vi "2_AdvancedDemo_TH260Histo.vi"() -> ()   [LabVIEW 2010]
uses:
  Types/TH260_UIThread_Cmds.ctl
  Types/TH260_UIThread_Data.ctl
  Types/TH260_InputChannel.ctl
  <vilib>/Utility/error.llb/DialogType.ctl
  _lib/PQ/TimeHarp260/th260lib_x86_x64_UIThread.llb/TH260_DllPath_global.vi
  _lib/PQ/TimeHarp260/TH260_LibVersion_global.vi
  _lib/PQ/TimeHarp260/TH260_InitInfo.ctl
  _lib/PQ/TimeHarp260/TH260_MeasMode.ctl
  _lib/PQ/TimeHarp260/TH260_TimingMode.ctl
panel:
  in  "Settings":bool=TRUE
  in  "Run continuously":bool=TRUE caption="Conti."
  in  "Start":bool
  in  "Scale":bool
  out "CountRates":i32[](graph)
  in  "HistoLength":i32(ring)=6 caption="Num Bins" items=["1024", "2048", "4096", "8192", "16384", "32768"]
  in  "OvlLevel":u32=100000 caption="Ovl.Level" min=1 step=1
  in  "StopOvl.":bool=TRUE
  in  "AcqTime":i32=1000 caption="Acqu.     ms" min=1 max=360000000 step=1
  in  "Binning":i32(ring) caption="Resol.      ps" items=["25", "50", "100", "200", "400", "800", "1600", "3200", "6400", "12800", "25600", "51200", "102400", "204800", "409600", "819200", "1638400", "3276800", "6553600", "13107200", "26214400", "52428800"]
  in  "HistoOffset":i32 caption="Offset      ns" min=0 max=100000000 step=1
  out "HistoGraph":T1(graph)={0.0, "Resolution"=0.001, "Histogram"=array8x1024[8192 elements]}
  in  "SyncTrgEdge":i32(ring) caption="Edge" items=["falling", "rising"]
  in  "SyncTrgLevel":i32=-100 caption="Level        mV" min=-1200 max=1200 step=1
  in  "SyncCFDLevel":i32=-100 caption="Level        mV" min=-1200 max=0 step=1
  in  "SyncZeroX":i32=-10 caption="ZeroCr.    mV" min=-40 max=0 step=1
  in  "SyncDivider":i32(ring)=3 caption="Divider" items=["1", "2", "4", "8"]
  in  "SyncOffset":i32 caption="Offset        ps" min=-99999 max=99999 step=1
  in  "Channels":T2[](array[typedef])=[{"Name"="Inp.Chan 1", "Enable"=TRUE, "Offset"=0, "CFDLevel"=50, "ZeroX"=10, "dtcode"=0, "TrgLevel"=-100, "TrgEdge"=0}, {"Name"="Inp.Chan 2", "Enable"=TRUE, "Offset"=0, "CFDLevel"=50, "ZeroX"=10, "dtcode"=0, "TrgLevel"=-100, "TrgEdge"=0}, {"Name"="Inp.Chan 3", "Enable"=TRUE, "Offset"=0, "CFDLevel"=50, "ZeroX"=10, "dtcode"=0, "TrgLevel"=-100, "TrgEdge"=0}, {"Name"="Inp.Chan 4", "Enable"=TRUE, "Offset"=0, "CFDLevel"=50, "ZeroX"=10, "dtcode"=0, "TrgLevel"=-100, "TrgEdge"=0}, {"Name"="Inp.Chan 5", "Enable"=TRUE, "Offset"=0, "CFDLevel"=50, "ZeroX"=10, "dtcode"=0, "TrgLevel"=-100, "TrgEdge"=0}, {"Name"="Inp.Chan 6", "Enable"=TRUE, "Offset"=0, "CFDLevel"=50, "ZeroX"=10, "dtcode"=0, "TrgLevel"=-100, "TrgEdge"=0}, {"Name"="Inp.Chan 7", "Enable"=TRUE, "Offset"=0, "CFDLevel"=50, "ZeroX"=10, "dtcode"=0, "TrgLevel"=-100, "TrgEdge"=0}, {"Name"="Inp.Chan 8", "Enable"=TRUE, "Offset"=0, "CFDLevel"=50, "ZeroX"=10, "dtcode"=0, "TrgLevel"=-100, "TrgEdge"=0}] {"TrgEdge" items=["falling", "rising"]; "TrgLevel" min=-1200 max=1200 step=1; "dtcode" items=["24", "44", "66", "88", "112", "135", "160", "180"]; "ZeroX" min=-40 max=0 step=1; "Offset" min=-99999 max=99999 step=1; "CFDLevel" min=-1200 max=0 step=1}
  out "SyncRate":string="Sync Rate: 0 cps\n"
  out "OverFlow":bool caption="Overflow:"
  out "Status":string="Initialized!"
  # "Histogram"
  # "Sync"
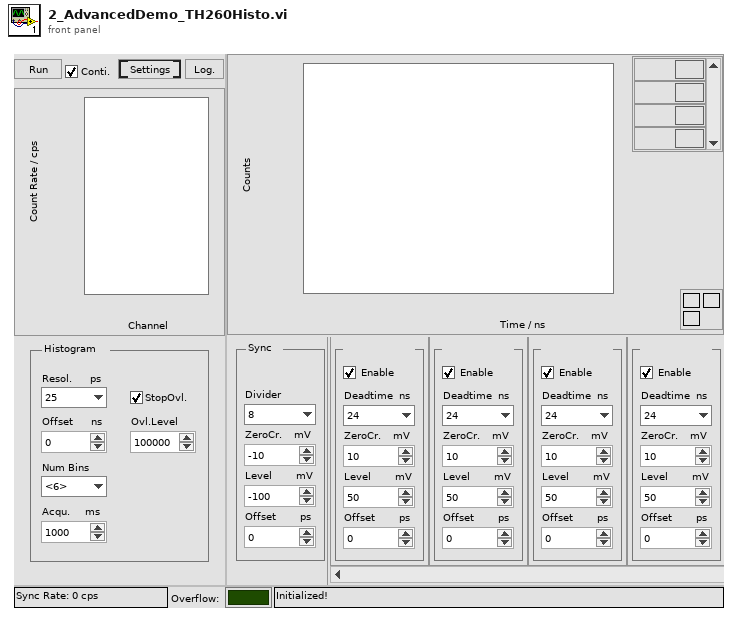
[diagram p1: front panel]
types:
  T1 = cluster{dbl, "Resolution":dbl, "Histogram":u32[][]}
  T2 = typedef "TH260_InputChannel.ctl" = cluster{"Name":string, "Enable":bool, "Offset":i32, "CFDLevel":i32, "ZeroX":i32, "dtcode":i32, "TrgLevel":i32, "TrgEdge":i32}
  T3 = typedef "TH260_UIThread_Data.ctl" = cluster{"Init Info":T4, "DevIdx":i32, "Channels":T2[], "CurrentChannels":i32[], "AcqTime":i32, "Binning":i32, "HistoOffset":i32, "HistoLen":i32, "StopOvl.":bool, "OvlLevel":u32, "StartMeas":bool, "HistoLength":i32, "Resolution":dbl, "Run cont.":bool, "Status":string, "SyncRate":i32, "BitShift":i32, "HistoAcqTime":dbl, "SyncTrgEdge":i32, "SyncTrgLevel":i32, "SyncCFDLevel":i32, "SyncZeroX":i32, "SyncDivider":i32, "SyncOffset":i32}
  T4 = typedef "TH260_InitInfo.ctl" = cluster{"Library Version":string, "Serial No.":string, "Model":string, "Partnum":string, "Version":string, "features":i32, "nchannels":i32, "Base Resolution":dbl, "Bin Steps":i32}
  T5 = typedef "TH260_UIThread_Cmds.ctl" = enum16{"Idle", "Init", "SetInpChanEnable", "SetInpChanOffset", "SetInpChanCFD", "SetInpChanTrg", "SetInpChanDeadtime", "SetSyncDivider", "SetSyncCFD", "SetSyncTrg", "SetSyncOffset", "SetBinning", "SetHistoOffset", "SetHistoLen", "SetStopOvl", "SetBitShift", "SetHistoAcqTime", "GetRates", "StartMeas", "StopMeas", "AbortMeas", "GetResolution", "GetHisto", "ReadFiFo", "WriteStatus", "Resize", "EnableControls", "DisableControls", "Error", "Exit"}
  T6 = enum8{"Enabled", "Disabled", "Disabled and Grayed Out"}
  T7 = typedef "TH260_TimingMode.ctl" = i32
  T8 = typedef "TH260_MeasMode.ctl" = i32
  T9 = typedef "DialogType.ctl" = u16
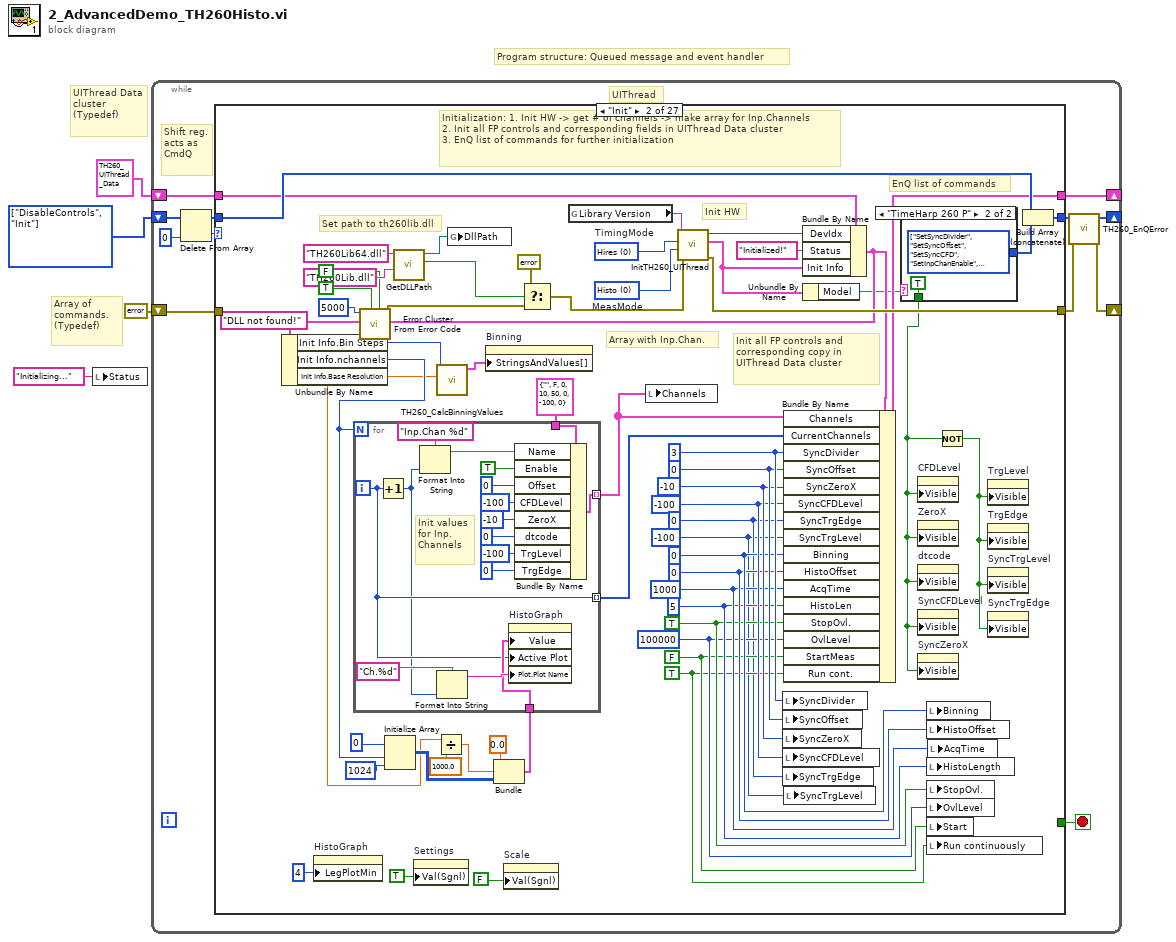
[diagram p0: block diagram]
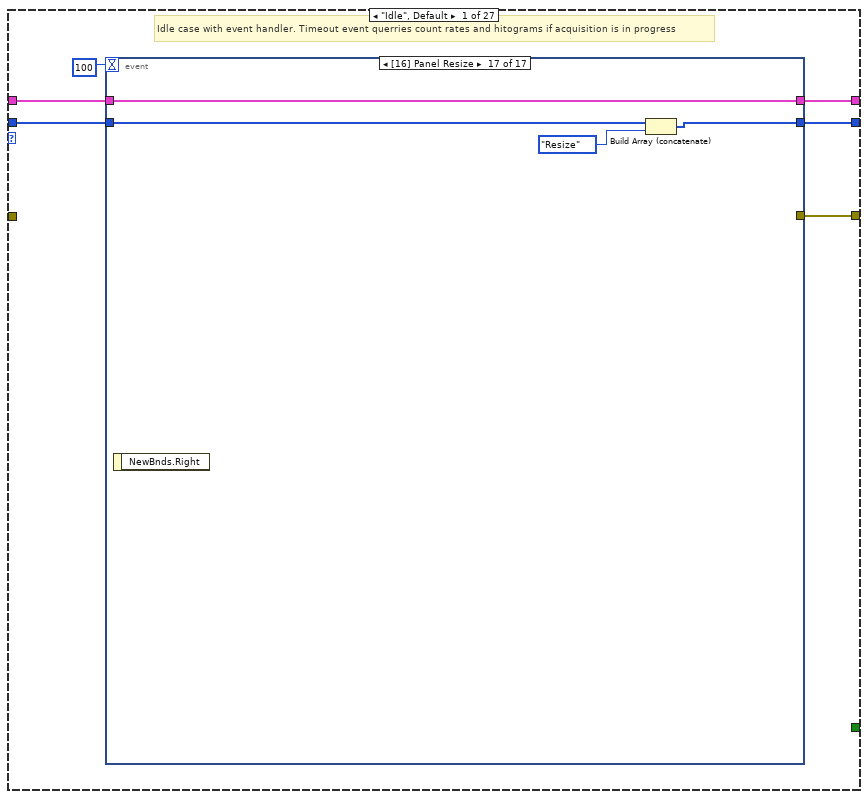
[diagram p2: hidden frame]
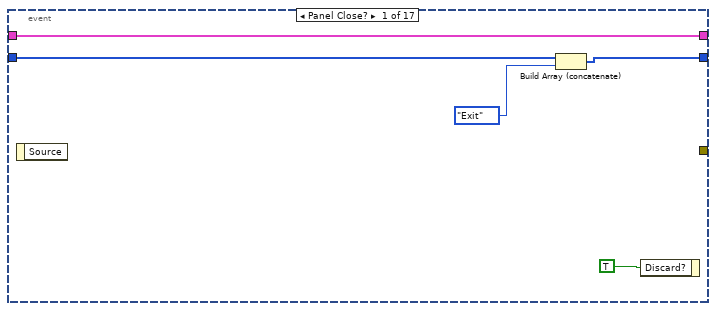
[diagram p3: hidden frame]
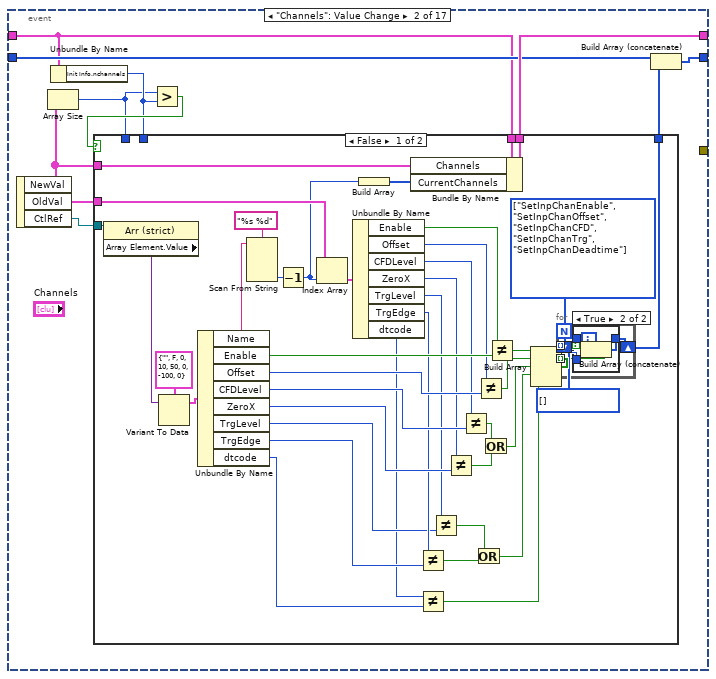
[diagram p4: hidden frame]
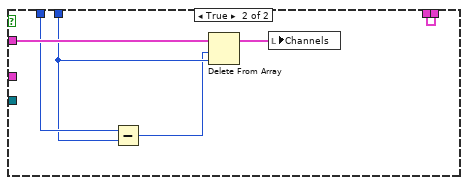
[diagram p6: hidden frame]
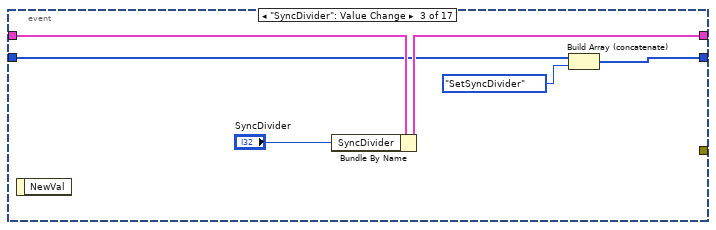
[diagram p7: hidden frame]
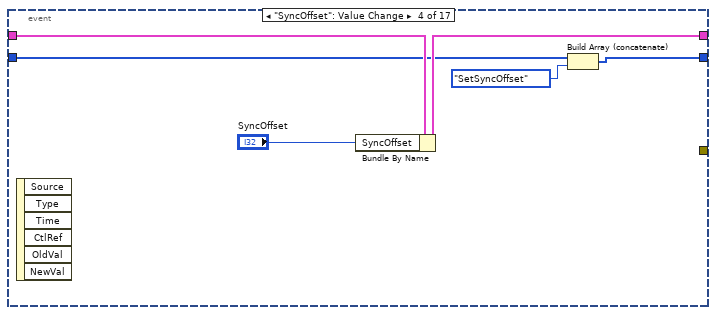
[diagram p8: hidden frame]
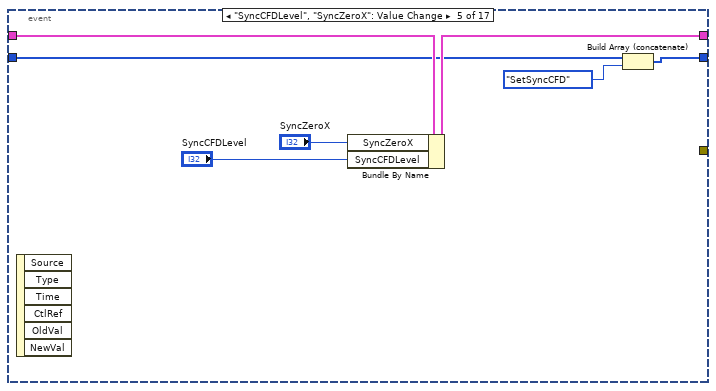
[diagram p9: hidden frame]
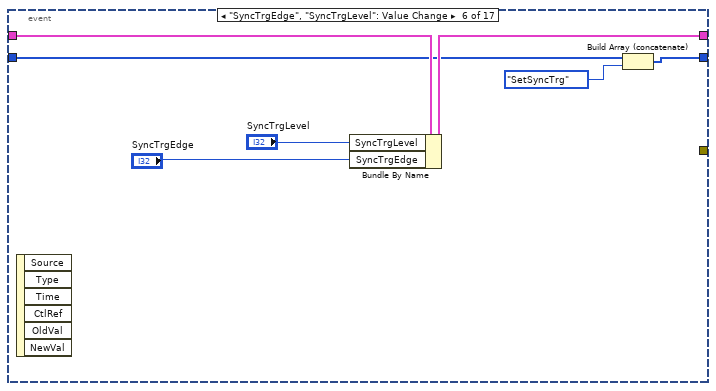
[diagram p10: hidden frame]
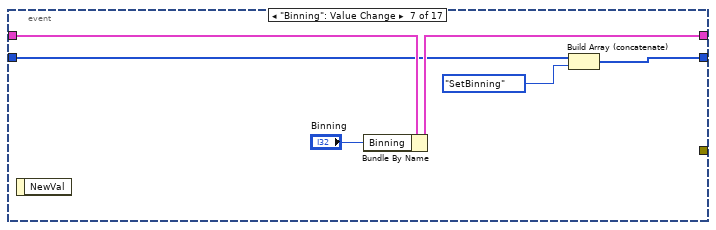
[diagram p11: hidden frame]
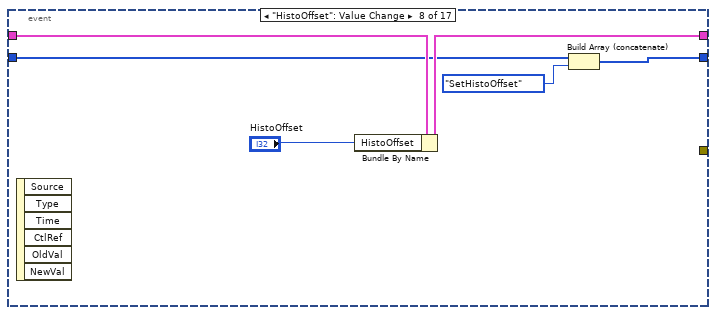
[diagram p12: hidden frame]
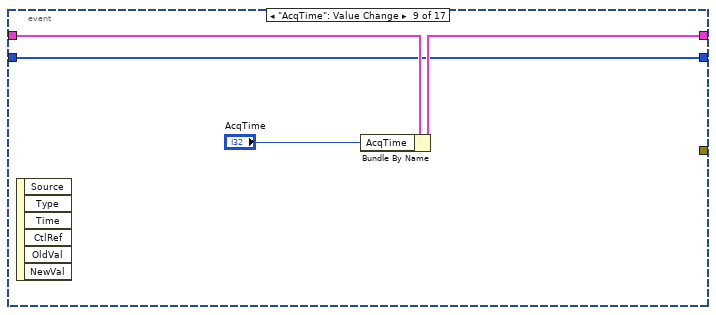
[diagram p13: hidden frame]
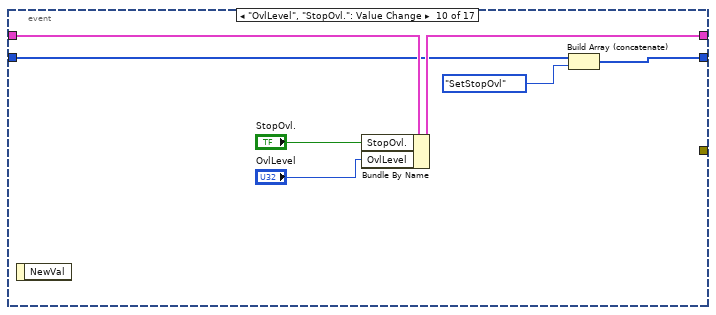
[diagram p14: hidden frame]
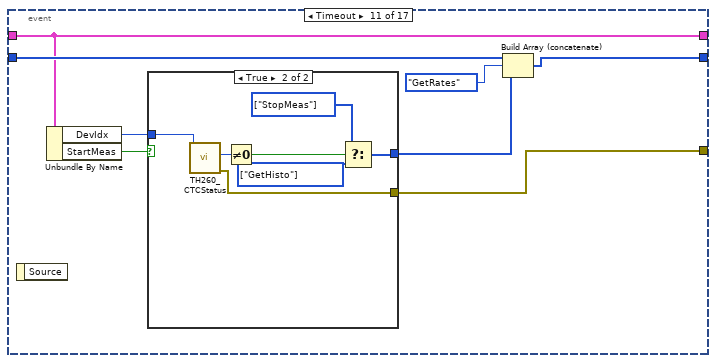
[diagram p15: hidden frame]
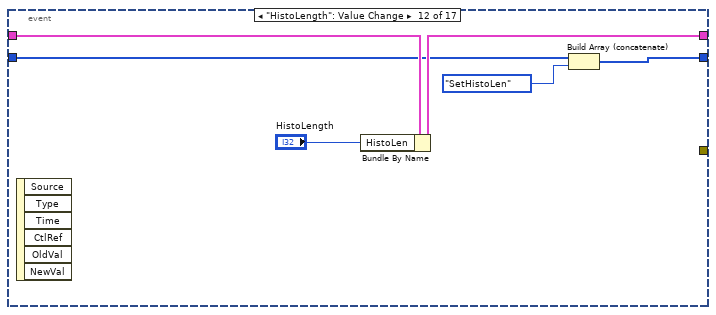
[diagram p17: hidden frame]
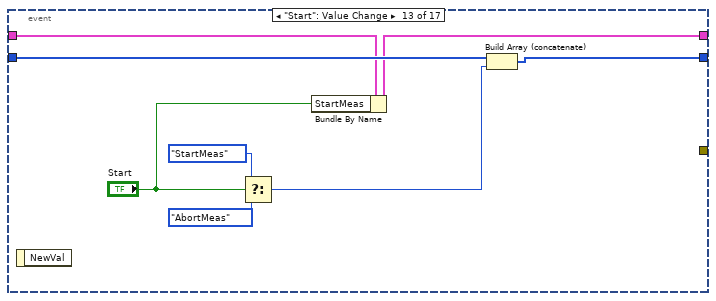
[diagram p18: hidden frame]
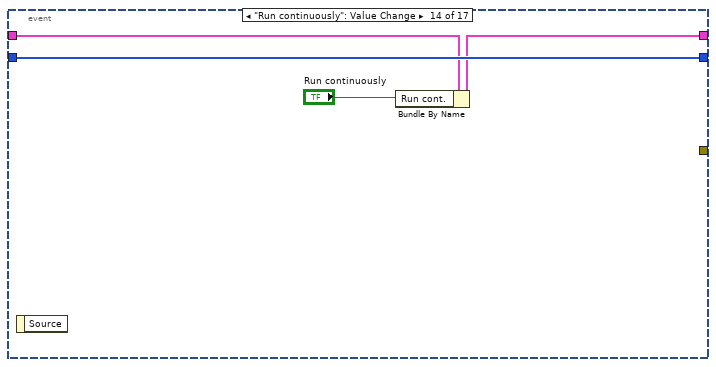
[diagram p19: hidden frame]
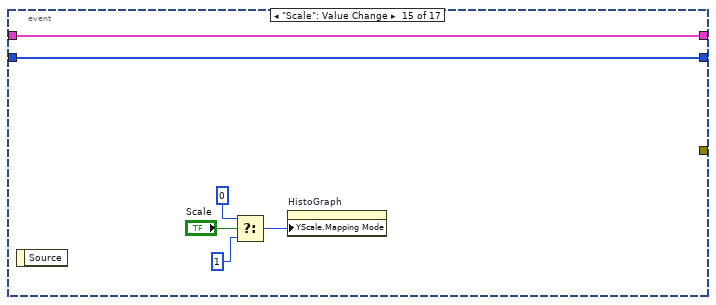
[diagram p20: hidden frame]
diagram:
  w3 = T5[] [enum."DisableControls", enum."Init"] items=["Idle", "Init", "SetInpChanEnable", "SetInpChanOffset", "SetInpChanCFD", "SetInpChanTrg", "SetInpChanDeadtime", "SetSyncDivider", "SetSyncCFD", "SetSyncTrg", "SetSyncOffset", "SetBinning", "SetHistoOffset", "SetHistoLen", "SetStopOvl", "SetBitShift", "SetHistoAcqTime", "GetRates", "StartMeas", "StopMeas", "AbortMeas", "GetResolution", "GetHisto", "ReadFiFo", "WriteStatus", "Resize", "EnableControls", "DisableControls", "Error", "Exit"]
  # "Array of commands.\n(Typedef)"
  # "Program structure: Queued message and event handler"
  # "UIThread Data cluster\n(Typedef)"
  n1 = local write "Status"("Initializing..." ("Status")) -> ()
  n2 = while {
    shift-right: [w5] -> _
    shift-left: w3 -> [w12]
    shift-right: [w15] -> _
    shift-left: T3 {"Init Info"={"Library Version"="", "Serial No."="", "Model"="", "Partnum"="", "Version"="", "features"=0, "nchannels"=0, "Base Resolution"=0.0, "Bin Steps"=0}, "DevIdx"=0, "Channels"=[], "CurrentChannels"=[], "AcqTime"=1, "Binning"=1, "HistoOffset"=1, "HistoLen"=1024, "StopOvl."=FALSE, "OvlLevel"=1024, "StartMeas"=FALSE, "HistoLength"=0, "Resolution"=0.0, "Run cont."=FALSE, "Status"="", "SyncRate"=0, "BitShift"=0, "HistoAcqTime"=0.0, "SyncTrgEdge"=0, "SyncTrgLevel"=-100, "SyncCFDLevel"=10, "SyncZeroX"=3, "SyncDivider"=3, "SyncOffset"=0} -> [w14]
    shift-right: [w7] -> _
    shift-left: errorcluster {"status"=FALSE, "code"=0, "source"=""} ("error IO") -> [w13]
    stop <- w16 stop-if-true
    # "Shift reg.\nacts as\nCmdQ"
    # "UIThread"
    n3 = Delete From Array(array=w12, index=0) -> (deleted portion=w10:T5, array with subset deleted=w9:T5[])  [unwired: 1 in]
    n4 = case shown="\"Init\"" w10 {
      tunnel: [w22 w256 w284 w298 w312 w327 w342 w358 w367 w373 w375 w382 w390 w398 w403 w415 w430 w438 w452 w466 w493 w518 w531 w538 w550 w556 w560] -> w6
      tunnel: [_ _ _ _ _ _ _ _ _ _ _ _ _ _ _ _ _ _ _ _ _ _ _ _ _ _ TRUE] -> w16
      tunnel: [w21 w236 w287 w301 w315 w330 w345 w360 w368 w374 w379 w386 w391 w393 w404 w414 w436 w441 w455 w462 w492 w517 w519 w537 w549 w557 w563] -> w15
      tunnel: w14 -> [w20 w241 w287 w301 w315 w330 w345 w360 w368 w374 w379 w386 w391 w394 w404 w414 w436 w442 w456 w463 w492 w517 w519 w537 w549 w557 w563]
      tunnel: [w17 w258 w285 w299 w313 w328 w343 w356 w366 w372 w378 w385 w389 w397 w402 w413 w435 w444 w458 w464 w488 _ _ _ _ _ w561] -> w8
      tunnel: w13 -> [_ _ _ _ _ _ _ _ _ _ _ _ _ _ _ _ _ _ _ _ _ _ _ _ _ w558 _]
      tunnel: w9 -> [w19 w257 w284 w298 w312 w327 w342 w358 w367 w373 w375 w381 w390 w398 w403 w415 w431 w439 w453 w466 w493 w518 w531 w538 w550 _ w560]
      frame "Idle", Default {
        # "Idle case with event handler. Timeout event querries count rates and hitograms if acquisition is in progress"
        n5 = event shown="[16] Panel Resize" {
          selector: _ -> [_ _ _ _ _ _ _ _ _ _ _ _ _ _ _ _ _]
          dyn-events: _ -> [_ _ _ _ _ _ _ _ _ _ _ _ _ _ _ _ _]
          timeout: 100 -> [_ _ _ _ _ _ _ _ _ _ _ _ _ _ _ _ _]
          tunnel: [w23 w33 w95 w101 w108 w115 w121 w127 w132 w138 w148 w159 w167 w175 w181 w189 w199] -> w22
          tunnel: [w26 w36 w98 w104 w111 w118 w124 w130 w134 w141 w147 w162 w165 w173 w180 w188 w202] -> w21
          tunnel: w20 -> [w26 w32 w99 w105 w112 w119 w125 w131 w135 w142 w147 w163 w166 w174 w180 w188 w202]
          tunnel: w19 -> [w25 w35 w97 w103 w110 w117 w123 w129 w132 w140 w150 w161 w169 w175 w181 w189 w200]
          tunnel: [_ _ _ _ _ _ _ _ _ _ w143 _ _ _ _ _ _] -> w17
          event Panel Close? {
            n6 = event-data() -> ()  [unwired: 1 in, 1 out]
            n7 = Build Array (concatenate)(w25, TH260_UIThread_Cmds."Exit") -> (w23:T5[])
            n8 = event-data("Discard?"=TRUE) -> ()  [unwired: 1 in, 1 out]
          }
          event "Channels": Value Change {
            n9 = event-data() -> ("NewVal"=w31:T2[], "OldVal"=w37:T2[], "CtlRef"=w38:refnum<vi>)  [unwired: 1 in]
            n10 = Array Size(array=w31) -> (size(s)=w28:i32)
            n11 = Unbundle By Name(w32) -> ("Init Info.nchannels"=w29:i32)
            n12 = Greater?(x=w28, y=w29) -> (0:w30:bool)
            n13 = case shown="False" w30 {
              tunnel: w38 -> [w79 _]
              tunnel: w37 -> [w73 _]
              tunnel: [w56 w93] -> w36
              tunnel: [w54 _] -> w34
              tunnel: w32 -> [w51 w93]
              tunnel: w31 -> [w50 w92]
              tunnel: w29 -> [_ w90]
              tunnel: w28 -> [_ w91]
              frame False {
                w39 = T5[] [] items=["Idle", "Init", "SetInpChanEnable", "SetInpChanOffset", "SetInpChanCFD", "SetInpChanTrg", "SetInpChanDeadtime", "SetSyncDivider", "SetSyncCFD", "SetSyncTrg", "SetSyncOffset", "SetBinning", "SetHistoOffset", "SetHistoLen", "SetStopOvl", "SetBitShift", "SetHistoAcqTime", "GetRates", "StartMeas", "StopMeas", "AbortMeas", "GetResolution", "GetHisto", "ReadFiFo", "WriteStatus", "Resize", "EnableControls", "DisableControls", "Error", "Exit"] ("Array")
                w57 = T5[] [enum."SetInpChanEnable", enum."SetInpChanOffset", enum."SetInpChanCFD", enum."SetInpChanTrg", enum."SetInpChanDeadtime"] items=["Idle", "Init", "SetInpChanEnable", "SetInpChanOffset", "SetInpChanCFD", "SetInpChanTrg", "SetInpChanDeadtime", "SetSyncDivider", "SetSyncCFD", "SetSyncTrg", "SetSyncOffset", "SetBinning", "SetHistoOffset", "SetHistoLen", "SetStopOvl", "SetBitShift", "SetHistoAcqTime", "GetRates", "StartMeas", "StopMeas", "AbortMeas", "GetResolution", "GetHisto", "ReadFiFo", "WriteStatus", "Resize", "EnableControls", "DisableControls", "Error", "Exit"]
                n14 = property class="Arr (strict)"(reference=w79) -> ("Array Element.Value"=w78:variant)  [unwired: 1 in, 2 out]
                n15 = Variant To Data(Variant=w78, type=T2 {"Name"="", "Enable"=FALSE, "Offset"=0, "CFDLevel"=10, "ZeroX"=50, "dtcode"=0, "TrgLevel"=-100, "TrgEdge"=0} ("Channel")) -> (data=w55:cluster{})  [unwired: 1 in, 1 out]
                n16 = Unbundle By Name(w55) -> ("Name"=w76:string, "Enable"=w70:bool, "Offset"=w68:i32, "CFDLevel"=w66:i32, "ZeroX"=w64:i32, "TrgLevel"=w47:i32, "TrgEdge"=w46:i32, "dtcode"=w41:i32)
                n17 = Scan From String(format string="%s %d", input string=w76) -> (output 2=w74:i32)  [unwired: 5 in, 3 out]
                n18 = Decrement(x=w74) -> (x-1=w53:i32)
                n19 = Index Array(array=w73, index=w53) -> (element=w72:T2)
                n20 = Unbundle By Name(w72) -> ("Enable"=w71:bool, "Offset"=w69:i32, "CFDLevel"=w67:i32, "ZeroX"=w65:i32, "TrgLevel"=w49:i32, "TrgEdge"=w48:i32, "dtcode"=w42:i32)
                n21 = Build Array(w53) -> (w52:i32[])
                n22 = Bundle By Name(cluster=w51, "Channels"=w50, "CurrentChannels"=w52) -> (w56:T3)
                n23 = Not Equal?(x=w48, y=w46) -> (x != y?=w44:bool)
                n24 = Not Equal?(x=w42, y=w41) -> (x != y?=w40:bool)
                n25 = Not Equal?(x=w49, y=w47) -> (x != y?=w45:bool)
                n26 = Not Equal?(x=w65, y=w64) -> (x != y?=w59:bool)
                n27 = Not Equal?(x=w67, y=w66) -> (x != y?=w60:bool)
                n28 = Or(x=w45, y=w44) -> (x .or. y?=w43:bool)
                n29 = Not Equal?(x=w69, y=w68) -> (x != y?=w62:bool)
                n30 = Or(x=w60, y=w59) -> (x .or. y?=w58:bool)
                n31 = Not Equal?(x=w71, y=w70) -> (x != y?=w63:bool)
                n32 = Build Array(w63, w62, w58, w43, w40) -> (w61:bool[])
                n33 = for {
                  tunnel: w61 -> [w82] mode=indexing
                  tunnel: w57 -> [w83] mode=indexing
                  shift-right: [w80] -> w54
                  shift-left: w39 -> [w81]
                  n34 = case shown="True" w82 {
                    tunnel: w81 -> [w84 w86]
                    tunnel: w83 -> [_ w85]
                    tunnel: [w84 w87] -> w80
                    frame False {
                    }
                    frame True {
                      n35 = Build Array (concatenate)(w86, w85) -> (w87:T5[])
                    }
                  }
                }
              }
              frame True {
                n36 = Subtract(x=w91, y=w90) -> (x-y=w89:i32)
                n37 = Delete From Array(array=w92, length=w89, index=w90) -> (array with subset deleted=w88:T2[])  [unwired: 1 out]
                n38 = local write "Channels"(w88) -> ()
              }
            }
            n39 = Build Array (concatenate)(w35, w34) -> (w33:T5[])
          }
          event "SyncDivider": Value Change {
            n40 = event-data() -> ()  [unwired: 1 in, 1 out]
            n41 = Bundle By Name(cluster=w99, "SyncDivider"="SyncDivider") -> (w98:T3)
            n42 = Build Array (concatenate)(w97, TH260_UIThread_Cmds."SetSyncDivider") -> (w95:T5[])
          }
          event "SyncOffset": Value Change {
            n43 = event-data() -> ()  [unwired: 1 in, 6 out]
            n44 = Bundle By Name(cluster=w105, "SyncOffset"="SyncOffset") -> (w104:T3)
            n45 = Build Array (concatenate)(w103, TH260_UIThread_Cmds."SetSyncOffset") -> (w101:T5[])
          }
          event "SyncCFDLevel", "SyncZeroX": Value Change {
            n46 = event-data() -> ()  [unwired: 1 in, 6 out]
            n47 = Bundle By Name(cluster=w112, "SyncZeroX"="SyncZeroX", "SyncCFDLevel"="SyncCFDLevel") -> (w111:T3)
            n48 = Build Array (concatenate)(w110, TH260_UIThread_Cmds."SetSyncCFD") -> (w108:T5[])
          }
          event "SyncTrgEdge", "SyncTrgLevel": Value Change {
            n49 = event-data() -> ()  [unwired: 1 in, 6 out]
            n50 = Bundle By Name(cluster=w119, "SyncTrgLevel"="SyncTrgLevel", "SyncTrgEdge"="SyncTrgEdge") -> (w118:T3)
            n51 = Build Array (concatenate)(w117, TH260_UIThread_Cmds."SetSyncTrg") -> (w115:T5[])
          }
          event "Binning": Value Change {
            n52 = event-data() -> ()  [unwired: 1 in, 1 out]
            n53 = Bundle By Name(cluster=w125, "Binning"="Binning") -> (w124:T3)
            n54 = Build Array (concatenate)(w123, TH260_UIThread_Cmds."SetBinning") -> (w121:T5[])
          }
          event "HistoOffset": Value Change {
            n55 = event-data() -> ()  [unwired: 1 in, 6 out]
            n56 = Bundle By Name(cluster=w131, "HistoOffset"="HistoOffset") -> (w130:T3)
            n57 = Build Array (concatenate)(w129, TH260_UIThread_Cmds."SetHistoOffset") -> (w127:T5[])
          }
          event "AcqTime": Value Change {
            n58 = event-data() -> ()  [unwired: 1 in, 6 out]
            n59 = Bundle By Name(cluster=w135, "AcqTime"="AcqTime") -> (w134:T3)
          }
          event "OvlLevel", "StopOvl.": Value Change {
            n60 = event-data() -> ()  [unwired: 1 in, 1 out]
            n61 = Bundle By Name(cluster=w142, "StopOvl."="StopOvl.", "OvlLevel"="OvlLevel") -> (w141:T3)
            n62 = Build Array (concatenate)(w140, TH260_UIThread_Cmds."SetStopOvl") -> (w138:T5[])
          }
          event Timeout {
            n63 = event-data() -> ()  [unwired: 1 in, 1 out]
            n64 = Unbundle By Name(w147) -> ("DevIdx"=w145:i32, "StartMeas"=w146:bool)
            n65 = case shown="True" w146 {
              tunnel: w145 -> [_ w157]
              tunnel: [_ w155] -> w144
              tunnel: [_ w152] -> w143
              frame False {
              }
              frame True {
                w153 = T5[] [enum."GetHisto"] items=["Idle", "Init", "SetInpChanEnable", "SetInpChanOffset", "SetInpChanCFD", "SetInpChanTrg", "SetInpChanDeadtime", "SetSyncDivider", "SetSyncCFD", "SetSyncTrg", "SetSyncOffset", "SetBinning", "SetHistoOffset", "SetHistoLen", "SetStopOvl", "SetBitShift", "SetHistoAcqTime", "GetRates", "StartMeas", "StopMeas", "AbortMeas", "GetResolution", "GetHisto", "ReadFiFo", "WriteStatus", "Resize", "EnableControls", "DisableControls", "Error", "Exit"]
                w154 = T5[] [enum."StopMeas"] items=["Idle", "Init", "SetInpChanEnable", "SetInpChanOffset", "SetInpChanCFD", "SetInpChanTrg", "SetInpChanDeadtime", "SetSyncDivider", "SetSyncCFD", "SetSyncTrg", "SetSyncOffset", "SetBinning", "SetHistoOffset", "SetHistoLen", "SetStopOvl", "SetBitShift", "SetHistoAcqTime", "GetRates", "StartMeas", "StopMeas", "AbortMeas", "GetResolution", "GetHisto", "ReadFiFo", "WriteStatus", "Resize", "EnableControls", "DisableControls", "Error", "Exit"]
                n66 = call "TH260_CTCStatus.vi"("devidx"=w157) -> ("error out"=w152:errorcluster, "ctcstatus"=w156:i32)  [unwired: 8 in, 1 out]
                n67 = Not Equal To 0?(x=w156) -> (x != 0?=w151:bool)
                n68 = Select(t=w154, s=w151, f=w153) -> (s? t:f=w155:T5[])
              }
            }
            n69 = Build Array (concatenate)(w150, TH260_UIThread_Cmds."GetRates", w144) -> (w148:T5[])
          }
          event "HistoLength": Value Change {
            n70 = event-data() -> ()  [unwired: 1 in, 6 out]
            n71 = Bundle By Name(cluster=w163, "HistoLen"="HistoLength") -> (w162:T3)
            n72 = Build Array (concatenate)(w161, TH260_UIThread_Cmds."SetHistoLen") -> (w159:T5[])
          }
          event "Start": Value Change {
            n73 = event-data() -> ()  [unwired: 1 in, 1 out]
            n74 = Select(t=TH260_UIThread_Cmds."StartMeas", s="Start", f=TH260_UIThread_Cmds."AbortMeas") -> (s? t:f=w168:T5)
            n75 = Bundle By Name(cluster=w166, "StartMeas"="Start") -> (w165:T3)
            n76 = Build Array (concatenate)(w169, w168) -> (w167:T5[])
          }
          event "Run continuously": Value Change {
            n77 = event-data() -> ()  [unwired: 1 in, 1 out]
            n78 = Bundle By Name(cluster=w174, "Run cont."="Run continuously") -> (w173:T3)
          }
          event "Scale": Value Change {
            n79 = event-data() -> ()  [unwired: 1 in, 1 out]
            n80 = Select(t=u8 0 ("Y Scale.Mapping Mode"), s="Scale", f=u8 1 ("Y Scale.Mapping Mode")) -> (s? t:f=w176:u8)
            n81 = property on="HistoGraph" class="WFGraph (strict)"("YScale.Mapping Mode"=w176) -> ()  [unwired: 2 in, 2 out]
          }
          event "Settings": Value Change {
            n82 = event-data() -> ()  [unwired: 1 in, 1 out]
            n83 = property on="Splitter" class="Splitter"() -> ("Position"=w187:i32)  [unwired: 2 in, 2 out]
            n84 = Select(t=250 ("PosT"), s="Settings", f=0 ("PosF")) -> (s? t:f=w184:i32)
            n85 = Subtract(x=w187, y=w184) -> (x-y=w183:i32)
            n86 = while {
              shift-right: [w198] -> _
              shift-left: w183 -> [w191]
              i -> [w197]
              stop <- w194 stop-if-true
              n87 = property on="Splitter 4" class="Splitter"("Position"=w191) -> (error out=w190:errorcluster)  [unwired: 2 in, 1 out]
              n88 = Greater Or Equal?(x=w197, y=10) -> (x >= y?=w195:bool)
              n89 = Decrement(x=w191) -> (x-1=w198:i32)
              n90 = Unbundle(w190) -> ("status"=w193:bool)  [unwired: 2 out]
              n91 = Not(x=w193) -> (.not. x?=w192:bool)
              n92 = Or(x=w192, y=w195) -> (x .or. y?=w194:bool)
            }
          }
          event Panel Resize {
            n93 = event-data() -> ()  [unwired: 1 in, 1 out]
            n94 = Build Array (concatenate)(w200, TH260_UIThread_Cmds."Resize") -> (w199:T5[])
          }
        }
      }
      frame "Init" {
        w209 = -100 ("SyncTrgLevel")
        w210 = 0 ("SyncTrgEdge")
        w215 = T7 0 items=["Hires", "Lowres"]  # TimingMode
        w216 = T8 0 items=["Histo"=0, "T2"=2, "T3"=3]  # MeasMode
        w243 = TRUE ("Run cont.")
        w245 = FALSE ("StartMeas")
        w246 = u32 100000 ("OvlLevel")
        w247 = TRUE ("StopOvl.")
        w248 = 5 ("HistoLen")
        w249 = 1000 ("AcqTime")
        w250 = 0 ("HistoOffset")
        w251 = 0 ("Binning")
        w252 = -100 ("SyncLevel")
        w253 = -10 ("SyncZeroX")
        w254 = 0 ("SyncOffset")
        w255 = 3 ("SyncDivider")
        # "Init HW"
        # "Set path to th260lib.dll"
        # "Init all FP controls and corresponding copy in UIThread Data cluster"
        # "EnQ list of commands"
        # "Array with Inp.Chan."
        # "Initialization: 1. Init HW -> get # of channels -> make array for Inp.Channels\n2. Init all FP controls and corresponding fields in UIThread Data cluster\n3. EnQ list of commands for further initialization"
        n95 = property on="HistoGraph" class="WFGraph (strict)"("LegPlotMin"=u32 4 ("Legend:Plot Minimum")) -> ()  [unwired: 2 in, 2 out]
        n96 = call <vilib>:"Error Cluster From Error Code.vi"("is warning? (False)"=FALSE, "show call chain? (False)"=TRUE, "error message (\"\")"="DLL not found!" ("error message (\"\")"), "error code (0)"=5000) -> ("error out"=w229:errorcluster)  [unwired: 5 in]
        n97 = call "GetDLLPath.vi"("DllName_32bit"="TH260Lib.dll" ("name or relative path"), "DllName_64bit"="TH260Lib64.dll" ("name or relative path")) -> ("file exists?"=w231:bool, "DLLPath"=w232:path)  [unwired: 8 in]
        n98 = property on="Settings" class="Bool (strict)"("Val(Sgnl)"=TRUE ("Value (Signaling)")) -> ()  [unwired: 2 in, 2 out]
        n99 = global write "TH260_DllPath_global.vi" "DllPath"(w232) -> ()
        n100 = property on="Scale" class="Bool (strict)"("Val(Sgnl)"=FALSE ("Value (Signaling)")) -> ()  [unwired: 2 in, 2 out]
        n101 = Select(t=errorcluster {"status"=FALSE, "code"=0, "source"=""} ("error IO"), s=w231, f=w229) -> (s? t:f=w237:errorcluster)
        n102 = global read "TH260_LibVersion_global.vi" "Library Version"() -> (w228:string)
        n103 = call "InitTH260_UIThread.vi"("error in (no error)"=w237, "MeasMode"=w216, "TimingMode"=w215, "Library Version"=w228) -> ("error out"=w258:errorcluster, "Init Info"=w214:T4, "DevIdx"=w260:i32)  [unwired: 5 in]
        n104 = local write "SyncDivider"(w255) -> ()
        n105 = local write "SyncOffset"(w254) -> ()
        n106 = local write "SyncZeroX"(w253) -> ()
        n107 = local write "SyncCFDLevel"(w252) -> ()
        n108 = local write "SyncTrgEdge"(w210) -> ()
        n109 = local write "SyncTrgLevel"(w209) -> ()
        n110 = Bundle By Name(cluster=w241, "DevIdx"=w260, "Status"="Initialized!", "Init Info"=w214) -> (w240:T3)
        n111 = Unbundle By Name(w240) -> ("Init Info.Bin Steps"=w239:i32, "Init Info.nchannels"=w218:i32, "Init Info.Base Resolution"=w208:dbl)
        n112 = Initialize Array(u32 0, w218, 1024 ("dimension size")) -> (w222:u32[][])
        n113 = Divide(x=w208, y=1000.0) -> (x/y=w223:dbl)
        n114 = call "TH260_CalcBinningValues.vi"("BaseRes"=w208, "Bin Steps"=w239) -> ("BinningValues"=w244:cluster{"String":string, "Value":i32}[])  [unwired: 9 in]
        n115 = property on="Binning" class="Ring (strict)"("StringsAndValues[]"=w244) -> ()  [unwired: 2 in, 2 out]
        n116 = Bundle(0.0, w223, w222) -> (w221:cluster{dbl, dbl, u32[][]})  [unwired: 1 in]
        n117 = for {
          N: w218 -> [_]
          tunnel: T2 {"Name"="", "Enable"=FALSE, "Offset"=0, "CFDLevel"=10, "ZeroX"=50, "dtcode"=0, "TrgLevel"=-100, "TrgEdge"=0} ("Channel") -> [w280]
          tunnel: [w279] -> w217 mode=indexing
          tunnel: [w269] -> w219 mode=indexing
          tunnel: w221 -> [w270]
          i -> [w269]
          # "Init values for Inp. Channels"
          n118 = Increment(x=w269) -> (x+1=w268:i32)
          n119 = Format Into String(format string="Inp.Chan %d", w268) -> (resulting string=w277:string)  [unwired: 2 in, 1 out]
          n120 = Format Into String(format string="Ch.%d", w268) -> (resulting string=w271:string)  [unwired: 2 in, 1 out]
          n121 = property on="HistoGraph" class="WFGraph (strict)"("Value"=w270, "Active Plot"=w269, "Plot.Plot Name"=w271) -> ()  [unwired: 2 in, 2 out]
          n122 = Bundle By Name(cluster=w280, "Name"=w277, "Enable"=TRUE, "Offset"=0, "CFDLevel"=-100 ("CFDZeroX"), "ZeroX"=-10 ("CFDLevel"), "dtcode"=0, "TrgLevel"=-100, "TrgEdge"=0) -> (w279:T2)
        }
        n123 = local write "Channels"(w217) -> ()
        n124 = Bundle By Name(cluster=w240, "Channels"=w217, "CurrentChannels"=w219, "SyncDivider"=w255, "SyncOffset"=w254, "SyncZeroX"=w253, "SyncCFDLevel"=w252, "SyncTrgEdge"=w210, "SyncTrgLevel"=w209, "Binning"=w251, "HistoOffset"=w250, "AcqTime"=w249, "HistoLen"=w248, "StopOvl."=w247, "OvlLevel"=w246, "StartMeas"=w245, "Run cont."=w243) -> (w236:T3)
        n125 = Unbundle By Name(w214) -> ("Model"=w213:string)
        n126 = case shown="\"TimeHarp 260 P\"" w213 {
          tunnel: [FALSE TRUE] -> w212
          tunnel: [w261 w263] -> w207
          frame Default {
            w261 = T5[] [enum."SetSyncDivider", enum."SetSyncOffset", enum."SetSyncTrg", enum."SetInpChanEnable", enum."SetInpChanOffset", enum."SetInpChanTrg", enum."SetBinning", enum."SetHistoOffset", enum."SetHistoLen", enum."SetStopOvl", enum."Resize", enum."EnableControls", enum."WriteStatus"] items=["Idle", "Init", "SetInpChanEnable", "SetInpChanOffset", "SetInpChanCFD", "SetInpChanTrg", "SetInpChanDeadtime", "SetSyncDivider", "SetSyncCFD", "SetSyncTrg", "SetSyncOffset", "SetBinning", "SetHistoOffset", "SetHistoLen", "SetStopOvl", "SetBitShift", "SetHistoAcqTime", "GetRates", "StartMeas", "StopMeas", "AbortMeas", "GetResolution", "GetHisto", "ReadFiFo", "WriteStatus", "Resize", "EnableControls", "DisableControls", "Error", "Exit"]
          }
          frame "TimeHarp 260 P" {
            w263 = T5[] [enum."SetSyncDivider", enum."SetSyncOffset", enum."SetSyncCFD", enum."SetInpChanEnable", enum."SetInpChanOffset", enum."SetInpChanCFD", enum."SetInpChanDeadtime", enum."SetBinning", enum."SetHistoOffset", enum."SetHistoLen", enum."SetStopOvl", enum."Resize", enum."EnableControls", enum."WriteStatus"] items=["Idle", "Init", "SetInpChanEnable", "SetInpChanOffset", "SetInpChanCFD", "SetInpChanTrg", "SetInpChanDeadtime", "SetSyncDivider", "SetSyncCFD", "SetSyncTrg", "SetSyncOffset", "SetBinning", "SetHistoOffset", "SetHistoLen", "SetStopOvl", "SetBitShift", "SetHistoAcqTime", "GetRates", "StartMeas", "StopMeas", "AbortMeas", "GetResolution", "GetHisto", "ReadFiFo", "WriteStatus", "Resize", "EnableControls", "DisableControls", "Error", "Exit"]
          }
        }
        n127 = property on="CFDLevel" class="DigNum (strict)"("Visible"=w212) -> ()  [unwired: 2 in, 2 out]
        n128 = property on="ZeroX" class="DigNum (strict)"("Visible"=w212) -> ()  [unwired: 2 in, 2 out]
        n129 = property on="dtcode" class="Ring (strict)"("Visible"=w212) -> ()  [unwired: 2 in, 2 out]
        n130 = property on="SyncCFDLevel" class="DigNum (strict)"("Visible"=w212) -> ()  [unwired: 2 in, 2 out]
        n131 = property on="SyncZeroX" class="DigNum (strict)"("Visible"=w212) -> ()  [unwired: 2 in, 2 out]
        n132 = local write "Binning"(w251) -> ()
        n133 = local write "HistoOffset"(w250) -> ()
        n134 = local write "HistoLength"(w248) -> ()
        n135 = local write "StopOvl."(w247) -> ()
        n136 = local write "OvlLevel"(w246) -> ()
        n137 = local write "Start"(w245) -> ()
        n138 = local write "Run continuously"(w243) -> ()
        n139 = local write "AcqTime"(w249) -> ()
        n140 = Not(x=w212) -> (.not. x?=w211:bool)
        n141 = property on="TrgLevel" class="DigNum (strict)"("Visible"=w211) -> ()  [unwired: 2 in, 2 out]
        n142 = property on="TrgEdge" class="Ring (strict)"("Visible"=w211) -> ()  [unwired: 2 in, 2 out]
        n143 = property on="SyncTrgLevel" class="DigNum (strict)"("Visible"=w211) -> ()  [unwired: 2 in, 2 out]
        n144 = property on="SyncTrgEdge" class="Ring (strict)"("Visible"=w211) -> ()  [unwired: 2 in, 2 out]
        n145 = Build Array (concatenate)(w257, w207) -> (w256:T5[])
      }
      frame "SetInpChanEnable" {
        n146 = Unbundle By Name(w287) -> ("DevIdx"=w286:i32, "Channels"=w281:T2[], "CurrentChannels"=w282:i32[])
        n147 = for {
          tunnel: w286 -> [w294]
          shift-right: [w293] -> w285
          shift-left: errorcluster {"status"=FALSE, "code"=0, "source"=""} ("error out") -> [w292]
          tunnel: w282 -> [w288] mode=indexing
          tunnel: w281 -> [w291]
          n148 = Index Array(array=w291, index=w288) -> (element=w290:T2)
          n149 = Unbundle By Name(w290) -> ("Enable"=w289:bool)
          n150 = call "TH260_SetInputChannelEnable.vi"("error in (no error)"=w292, "enable"=w289, "channel"=w288, "devidx"=w294) -> ("error out"=w293:errorcluster)  [unwired: 6 in, 1 out]
        }
      }
      frame "SetInpChanOffset" {
        n151 = Unbundle By Name(w301) -> ("DevIdx"=w300:i32, "Channels"=w295:T2[], "CurrentChannels"=w296:i32[])
        n152 = for {
          tunnel: w300 -> [w306]
          shift-right: [w303] -> w299
          shift-left: errorcluster {"status"=FALSE, "code"=0, "source"=""} ("error out") -> [w304]
          tunnel: w296 -> [w305] mode=indexing
          tunnel: w295 -> [w308]
          n153 = Index Array(array=w308, index=w305) -> (element=w307:T2)
          n154 = Unbundle By Name(w307) -> ("Offset"=w302:i32)
          n155 = call "TH260_SetInputChannelOffset.vi"("error in (no error)"=w304, "offset"=w302, "channel"=w305, "devidx"=w306) -> ("error out"=w303:errorcluster)  [unwired: 6 in, 1 out]
        }
      }
      frame "SetInpChanTrg" {
        n156 = Unbundle By Name(w315) -> ("DevIdx"=w314:i32, "Channels"=w309:T2[], "CurrentChannels"=w310:i32[])
        n157 = for {
          tunnel: w314 -> [w318]
          shift-right: [w320] -> w313
          shift-left: errorcluster {"status"=FALSE, "code"=0, "source"=""} ("error out") -> [w321]
          tunnel: w310 -> [w319] mode=indexing
          tunnel: w309 -> [w323]
          n158 = Index Array(array=w323, index=w319) -> (element=w322:T2)
          n159 = Unbundle By Name(w322) -> ("TrgLevel"=w317:i32, "TrgEdge"=w316:i32)
          n160 = call "TH260_SetInputEdgeTrg.vi"("channel"=w319, "error in (no error)"=w321, "edge"=w316, "level"=w317, "devidx"=w318) -> ("error out"=w320:errorcluster)  [unwired: 5 in, 1 out]
        }
      }
      frame "SetInpChanCFD" {
        n161 = Unbundle By Name(w330) -> ("DevIdx"=w329:i32, "Channels"=w324:T2[], "CurrentChannels"=w325:i32[])
        n162 = for {
          tunnel: w329 -> [w333]
          shift-right: [w335] -> w328
          shift-left: errorcluster {"status"=FALSE, "code"=0, "source"=""} ("error out") -> [w336]
          tunnel: w325 -> [w334] mode=indexing
          tunnel: w324 -> [w338]
          n163 = Index Array(array=w338, index=w334) -> (element=w337:T2)
          n164 = Unbundle By Name(w337) -> ("CFDLevel"=w332:i32, "ZeroX"=w331:i32)
          n165 = call "TH260_SetInputCFD.vi"("channel"=w334, "error in (no error)"=w336, "CFD ZeroCross"=w331, "CFD Level"=w332, "devidx"=w333) -> ("error out"=w335:errorcluster)  [unwired: 5 in, 1 out]
        }
      }
      frame "SetInpChanDeadtime" {
        n166 = Unbundle By Name(w345) -> ("DevIdx"=w344:i32, "Channels"=w339:T2[], "CurrentChannels"=w340:i32[])
        n167 = for {
          tunnel: w344 -> [w347]
          shift-right: [w349] -> w343
          shift-left: errorcluster {"status"=FALSE, "code"=0, "source"=""} ("error out") -> [w350]
          tunnel: w340 -> [w348] mode=indexing
          tunnel: w339 -> [w352]
          n168 = Index Array(array=w352, index=w348) -> (element=w351:T2)
          n169 = Unbundle By Name(w351) -> ("dtcode"=w346:i32)
          n170 = call "TH260_SetInputDeadTime.vi"("error in (no error)"=w350, "dtcode"=w346, "channel"=w348, "devidx"=w347) -> ("error out"=w349:errorcluster)  [unwired: 6 in, 1 out]
        }
      }
      frame "SetSyncDivider" {
        n171 = Unbundle By Name(w360) -> ("DevIdx"=w359:i32, "SyncDivider"=w355:i32)
        n172 = Power Of 2(x=w355) -> (2^x=w354:dbl)
        n173 = To Long Integer(number=w354) -> (32bit integer=w353:i32)
        n174 = call "TH260_SetSyncDiv.vi"("SyncDivider"=w353, "devidx"=w359) -> ("error out"=w357:errorcluster)  [unwired: 8 in, 1 out]
        n175 = flat-sequence {
          tunnel: w357 -> [w361]
          tunnel: [w361] -> w356
          frame #0 {
            n176 = Wait (ms)(milliseconds to wait=u32 100) -> ()  [unwired: 1 out]
          }
        }
      }
      frame "SetSyncTrg" {
        n177 = Unbundle By Name(w368) -> ("DevIdx"=w365:i32, "SyncTrgLevel"=w363:i32, "SyncTrgEdge"=w364:i32)
        n178 = call "TH260_SetSyncEdgeTrg.vi"("edge"=w364, "level"=w363, "devidx"=w365) -> ("error out"=w366:errorcluster)  [unwired: 7 in, 1 out]
      }
      frame "SetSyncCFD" {
        n179 = Unbundle By Name(w374) -> ("DevIdx"=w371:i32, "SyncCFDLevel"=w369:i32, "SyncZeroX"=w370:i32)
        n180 = call "TH260_SetSyncCFD.vi"("CFD ZeroCross"=w370, "CFD Level"=w369, "devidx"=w371) -> ("error out"=w372:errorcluster)  [unwired: 7 in, 1 out]
      }
      frame "SetSyncOffset" {
        n181 = Unbundle By Name(w379) -> ("DevIdx"=w377:i32, "SyncOffset"=w376:i32)
        n182 = call "TH260_SetSyncChannelOffset.vi"("Offset"=w376, "devidx"=w377) -> ("error out"=w378:errorcluster)  [unwired: 8 in, 1 out]
      }
      frame "SetBinning" {
        # "When binning is changed the new resolution is querried"
        n183 = Unbundle By Name(w386) -> ("DevIdx"=w384:i32, "Binning"=w383:i32)
        n184 = call "TH260_SetBinning.vi"("Binning"=w383, "devidx"=w384) -> ("error out"=w385:errorcluster)  [unwired: 8 in, 1 out]
        n185 = Build Array (concatenate)(TH260_UIThread_Cmds."GetResolution", w381) -> (w382:T5[])
      }
      frame "SetHistoOffset" {
        n186 = Unbundle By Name(w391) -> ("DevIdx"=w388:i32, "HistoOffset"=w387:i32)
        n187 = call "TH260_SetOffset.vi"("Offset"=w387, "devidx"=w388) -> ("error out"=w389:errorcluster)  [unwired: 8 in, 1 out]
      }
      frame "SetHistoLen" {
        n188 = Unbundle By Name(w394) -> ("DevIdx"=w396:i32, "HistoLen"=w395:i32)
        n189 = call "TH260_SetHistoLen.vi"("lencode"=w395, "devidx"=w396) -> ("error out"=w397:errorcluster, "actuallen"=w392:i32)  [unwired: 7 in, 1 out]
        n190 = Bundle By Name(cluster=w394, "HistoLength"=w392) -> (w393:T3)
      }
      frame "SetStopOvl" {
        n191 = Unbundle By Name(w404) -> ("DevIdx"=w401:i32, "StopOvl."=w400:bool, "OvlLevel"=w399:u32)
        n192 = call "TH260_SetStopOverflow.vi"("stopcount"=w399, "StopOnOverflow"=w400, "devidx"=w401) -> ("error out"=w402:errorcluster)  [unwired: 7 in, 1 out]
      }
      frame "GetRates" {
        n193 = Unbundle By Name(w414) -> ("Init Info.nchannels"=w412:i32, "Channels"=w405:T2[], "DevIdx"=w406:i32)
        n194 = call "TH260_GetSyncRate.vi"("devidx"=w406) -> ("error out"=w411:errorcluster, "rate"=w410:i32)  [unwired: 8 in, 1 out]
        n195 = Format Into String(format string="Sync Rate: %d cps\n", w410) -> (resulting string=→"SyncRate":string)  [unwired: 2 in, 1 out]
        n196 = for {
          N: w412 -> [_]
          tunnel: w406 -> [w421]
          tunnel: [w418] -> w408 mode=indexing
          shift-right: [w420] -> w413
          shift-left: w411 -> [w422]
          tunnel: w405 -> [w417] mode=indexing
          i -> [w419]
          n197 = Unbundle By Name(w417) -> ("Enable"=w416:bool)
          n198 = case shown="True" w416 {
            tunnel: w422 -> [w423 w428]
            tunnel: w421 -> [_ w427]
            tunnel: [w423 w426] -> w420
            tunnel: w419 -> [_ w425]
            tunnel: [_ w424] -> w418
            frame False {
            }
            frame True {
              n199 = call "TH260_GetCountRate.vi"("error in (no error)"=w428, "Channel"=w425, "devidx"=w427) -> ("error out"=w426:errorcluster, "rate"=w424:i32)  [unwired: 6 in, 1 out]
            }
          }
        }
        "CountRates" <- w408
      }
      frame "StartMeas" {
        n200 = Unbundle By Name(w436) -> ("AcqTime"=w432:i32, "DevIdx"=w433:i32)
        n201 = call "TH260_ClearHistMem.vi"("devidx"=w433) -> ("error out"=w434:errorcluster)  [unwired: 9 in, 1 out]
        n202 = call "TH260_StartMeas.vi"("error in (no error)"=w434, "Acquisition time"=w432, "devidx"=w433) -> ("error out"=w435:errorcluster)  [unwired: 7 in, 1 out]
        n203 = Build Array (concatenate)(w431, TH260_UIThread_Cmds."GetHisto") -> (w430:T5[])
      }
      frame "StopMeas" {
        n204 = Unbundle By Name(w442) -> ("Run cont."=w437:bool, "DevIdx"=w443:i32)
        n205 = call "TH260_StopMeas.vi"("devidx"=w443) -> ("error out"=w444:errorcluster)  [unwired: 9 in, 1 out]
        n206 = case shown="False" w437 {
          tunnel: w442 -> [w448 w450]
          tunnel: [w447 w450] -> w441
          tunnel: [w445 w449] -> w440
          frame False {
            w445 = T5[] [enum."GetHisto"] items=["Idle", "Init", "SetInpChanEnable", "SetInpChanOffset", "SetInpChanCFD", "SetInpChanTrg", "SetInpChanDeadtime", "SetSyncDivider", "SetSyncCFD", "SetSyncTrg", "SetSyncOffset", "SetBinning", "SetHistoOffset", "SetHistoLen", "SetStopOvl", "SetBitShift", "SetHistoAcqTime", "GetRates", "StartMeas", "StopMeas", "AbortMeas", "GetResolution", "GetHisto", "ReadFiFo", "WriteStatus", "Resize", "EnableControls", "DisableControls", "Error", "Exit"]
            w446 = FALSE ("StartMeas")
            n207 = Bundle By Name(cluster=w448, "StartMeas"=w446) -> (w447:T3)
            n208 = local write "Start"(w446) -> ()
          }
          frame True {
            w449 = T5[] [enum."GetHisto", enum."StartMeas"] items=["Idle", "Init", "SetInpChanEnable", "SetInpChanOffset", "SetInpChanCFD", "SetInpChanTrg", "SetInpChanDeadtime", "SetSyncDivider", "SetSyncCFD", "SetSyncTrg", "SetSyncOffset", "SetBinning", "SetHistoOffset", "SetHistoLen", "SetStopOvl", "SetBitShift", "SetHistoAcqTime", "GetRates", "StartMeas", "StopMeas", "AbortMeas", "GetResolution", "GetHisto", "ReadFiFo", "WriteStatus", "Resize", "EnableControls", "DisableControls", "Error", "Exit"]
          }
        }
        n209 = Build Array (concatenate)(w439, w440) -> (w438:T5[])
      }
      frame "AbortMeas" {
        w454 = T5[] [enum."GetHisto"] items=["Idle", "Init", "SetInpChanEnable", "SetInpChanOffset", "SetInpChanCFD", "SetInpChanTrg", "SetInpChanDeadtime", "SetSyncDivider", "SetSyncCFD", "SetSyncTrg", "SetSyncOffset", "SetBinning", "SetHistoOffset", "SetHistoLen", "SetStopOvl", "SetBitShift", "SetHistoAcqTime", "GetRates", "StartMeas", "StopMeas", "AbortMeas", "GetResolution", "GetHisto", "ReadFiFo", "WriteStatus", "Resize", "EnableControls", "DisableControls", "Error", "Exit"]
        w451 = FALSE ("StartMeas")
        n210 = Unbundle By Name(w456) -> ("DevIdx"=w457:i32)
        n211 = call "TH260_StopMeas.vi"("devidx"=w457) -> ("error out"=w458:errorcluster)  [unwired: 9 in, 1 out]
        n212 = Bundle By Name(cluster=w456, "StartMeas"=w451) -> (w455:T3)
        n213 = local write "Start"(w451) -> ()
        n214 = Build Array (concatenate)(w453, w454) -> (w452:T5[])
      }
      frame "GetResolution" {
        # "Resolution in ns"
        # "Gets resolution in ps"
        # "Resolution is saved in UIThread Data cluster in ns"
        n215 = Unbundle By Name(w463) -> ("DevIdx"=w465:i32)
        n216 = call "TH260_GetResolution.vi"("devidx"=w465) -> ("error out"=w464:errorcluster, "resolution"=w461:dbl)  [unwired: 8 in, 1 out]
        n217 = Divide(x=w461, y=1000.0) -> (x/y=w459:dbl)
        n218 = Bundle By Name(cluster=w463, "Resolution"=w459) -> (w462:T3)
      }
      frame "GetHisto" {
        w477 = 1  # FLAG_OVERFLOW
        # "Provides a buffer (U32-array of length 'HistoLength') for histograms."
        n219 = Unbundle By Name(w492) -> ("Resolution"=w489:dbl, "Init Info.nchannels"=w469:i32, "Channels"=w470:T2[], "DevIdx"=w491:i32, "HistoLength"=w490:i32)
        n220 = call "TH260_AllocateHistoBuffer.vi"("HistoLength"=w490) -> ("Buffer"=w483:u32[])  [unwired: 10 in]
        n221 = property class="VI"() -> ("Panel"=w468:refnum<vi>)  [unwired: 2 in, 2 out]
        n222 = for {
          N: w469 -> [_]
          tunnel: w491 -> [w506]
          tunnel: [w503] -> w480 mode=indexing
          tunnel: w483 -> [w504]
          shift-right: [w505] -> w479
          shift-left: errorcluster {"status"=FALSE, "code"=0, "source"=""} ("error IO") -> [w497]
          shift-right: [w498] -> w472
          shift-left: "Total Counts:\t\t" -> [w496]
          tunnel: w470 -> [w495] mode=indexing
          i -> [w502]
          n223 = Unbundle By Name(w495) -> ("Enable"=w494:bool)
          n224 = case shown="True" w494 {
            tunnel: w506 -> [_ w515]
            tunnel: [w507 w514] -> w505
            tunnel: w504 -> [w508 w513]
            tunnel: [w508 w512] -> w503
            tunnel: w502 -> [_ w511]
            tunnel: w497 -> [w507 w510]
            frame False {
            }
            frame True {
              n225 = call "TH260_GetHistogram.vi"("devidx"=w515, "Buffer"=w513, "clear"=FALSE, "error in (no error)"=w510, "channel"=w511) -> ("Histogram"=w512:u32[], "error out"=w514:errorcluster)  [unwired: 3 in, 1 out]
            }
          }
          n226 = Add Array Elements(numeric array=w503) -> (sum=w499:u32)
          n227 = Increment(x=w502) -> (x+1=w500:i32)
          n228 = Format Into String(format string="Ch.%2d: %d cnts.\t\t", initial string=w496, w500, w499) -> (resulting string=w498:string)  [unwired: 1 in, 1 out]
        }
        n229 = property class="Pnl"(reference=w468, "DeferPanUpdts"=FALSE ("Defer Panel Updates")) -> ()  [unwired: 1 in, 2 out]
        n230 = call "CalcRate.vi"("Refresh(ms)"=u32 500) -> ("Rate / Hz"=w487:dbl)  [unwired: 8 in, 2 out]
        n231 = Format Into String(format string="Readout Rate: %.1f Hz\\t\\t", w487) -> (resulting string=w485:string)  [unwired: 2 in, 1 out]
        n232 = Concatenate Strings(w485, w472) -> (w484:string)
        n233 = Bundle(0.0, "Resolution"=w489, "Histogram"=w480) -> (→"HistoGraph":T1)  [unwired: 1 in]
        n234 = local write "Status"(w484) -> ()
        n235 = call "TH260_GetFlags.vi"("error in (no error)"=w479) -> ("error out"=w488:errorcluster, "flags"=w476:i32)  [unwired: 8 in, 1 out]
        n236 = And(x=w477, y=w476) -> (x .and. y?=w478:i32)
        n237 = Not Equal To 0?(x=w478) -> (x != 0?=→"OverFlow":bool)
      }
      frame "WriteStatus" {
        n238 = Unbundle By Name(w517) -> ("Status"=→"Status":string)
      }
      frame "Resize" {
        n239 = property on="Pane 3" class="Pane"() -> ("Width"=w524:u32)  [unwired: 2 in, 2 out]
        n240 = Subtract(x=w524, y=i16 100 ("b")) -> (x-y=w530:u32)
        n241 = Unbundle By Name(w519) -> ("Init Info.nchannels"=w527:i32)
        n242 = Quotient & Remainder(x=w530, y=i16 99 ("m")) -> (floor(x/y)=w529:u32)  [unwired: 1 out]
        n243 = In Range and Coerce(upper limit=w527, x=w529, lower limit=4) -> (coerced(x)=w528:u32)  [unwired: 1 out]
        n244 = Equal?(x=w527, y=w528) -> (x = y?=w526:bool)
        n245 = Not(x=w526) -> (.not. x?=w525:bool)
        n246 = property on="Channels" class="Arr (strict)"("HorizScroll"=w525, "Number of Columns"=w528, "Index Values"=u32[] [0]) -> ()  [unwired: 2 in, 2 out]
      }
      frame "EnableControls" {
        n247 = property class="VI"() -> ("Panel"=w535:refnum<vi>)  [unwired: 2 in, 2 out]
        n248 = property class="Pnl"(reference=w535) -> ("Controls[]"=w534:refnum<vi>[])  [unwired: 1 in, 2 out]
        n249 = property class="Pnl"(reference=w535) -> ("Decos[]"=w536:refnum<vi>[])  [unwired: 1 in, 2 out]
        n250 = for {
          tunnel: w536 -> [w540] mode=indexing
          tunnel: TRUE -> [w539]
          n251 = property class="Decor"(reference=w540, "Visible"=w539) -> ()  [unwired: 1 in, 2 out]
        }
        n252 = for {
          tunnel: w534 -> [w543] mode=indexing
          tunnel: T6."Enabled" ("Disabled") -> [w542]
          tunnel: [w541] -> _
          n253 = property class="Ctl"(reference=w543, "DisabledEnum"=w542) -> (error out=w541:errorcluster)  [unwired: 1 in, 1 out]
        }
      }
      frame "DisableControls" {
        n254 = property class="VI"() -> ("Panel"=w547:refnum<vi>)  [unwired: 2 in, 2 out]
        n255 = property class="Pnl"(reference=w547) -> ("Controls[]"=w546:refnum<vi>[])  [unwired: 1 in, 2 out]
        n256 = property class="Pnl"(reference=w547) -> ("Decos[]"=w548:refnum<vi>[])  [unwired: 1 in, 2 out]
        n257 = for {
          tunnel: w548 -> [w552] mode=indexing
          tunnel: FALSE -> [w551]
          n258 = property class="Decor"(reference=w552, "Visible"=w551) -> ()  [unwired: 1 in, 2 out]
        }
        n259 = for {
          tunnel: w546 -> [w555] mode=indexing
          tunnel: T6."Disabled and Grayed Out" ("Disabled") -> [w554]
          tunnel: [w553] -> _
          n260 = property class="Ctl"(reference=w555, "DisabledEnum"=w554) -> (error out=w553:errorcluster)  [unwired: 1 in, 1 out]
        }
      }
      frame "Error" {
        w556 = T5[] [enum."Exit"] items=["Idle", "Init", "SetInpChanEnable", "SetInpChanOffset", "SetInpChanCFD", "SetInpChanTrg", "SetInpChanDeadtime", "SetSyncDivider", "SetSyncCFD", "SetSyncTrg", "SetSyncOffset", "SetBinning", "SetHistoOffset", "SetHistoLen", "SetStopOvl", "SetBitShift", "SetHistoAcqTime", "GetRates", "StartMeas", "StopMeas", "AbortMeas", "GetResolution", "GetHisto", "ReadFiFo", "WriteStatus", "Resize", "EnableControls", "DisableControls", "Error", "Exit"]
        w559 = T9 1 items=["no dialog", "OK message", "continue or stop message", "OK message + warnings", "continue/stop + warnings"] ("type of dialog (OK msg:1)")
        # "Error case: If an error occures the user is informed and the programm terminates. Add your own code to handle error events (e.g. exception lists, etc.)"
        n261 = call <vilib>:"Simple Error Handler.vi"("type of dialog (OK msg:1)"=w559, "error in (no error)"=w558) -> ()  [unwired: 3 in, 5 out]
      }
      frame "Exit" {
        n262 = Unbundle By Name(w563) -> ("DevIdx"=w562:i32)
        n263 = call "TH260_CloseDevice.vi"("devidx"=w562) -> ("error out"=w561:errorcluster)  [unwired: 9 in, 1 out]
      }
    }
    n264 = call "TH260_EnQError.vi"("error in (no error)"=w8, "Cmds_in"=w6) -> ("error out"=w7:errorcluster, "Cmds_out"=w5:T5[])  [unwired: 8 in]
  }
